vi "JTAG Function.vi"(0 "Enum":T1(ring)=enum."MULTI_ADC12_REPEAT", 1 "ARG 4":u16 format="%04x", 2 "ARG 5":u16 format="%04x", 3 "ARG 6":u16 format="%04x", 5 "ARG 1":u16 format="%04x", 7 "ARG 2":u16 format="%04x", 9 "ARG 3":u16 format="%04x", 11 "error in (no error)":errorcluster) -> (4 "ARG 7":u16 format="%04x", 8 "ARG1-ARG7":u16[](array[numeric]) format="%04x", 15 "error out":errorcluster)   [LabVIEW 2010]
panel:
  # "ARG1"
  # "ARG2"
  # "ARG3"
  # "ARG4"
  # "ARG5"
  # "ARG6"
  # "ARG7"
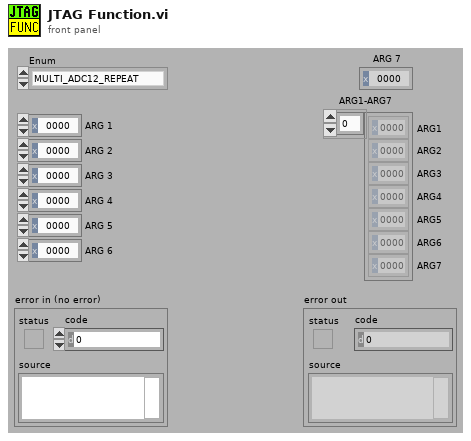
[diagram p1: front panel]
types:
  T1 = enum8{"PORT_OUT", "PORT_SEL", "PORT_RES_EN", "READ_PORT", "PORT_DIR", "SET_LCM", "PLUTO_WRITE_SINGLE", "PLUTO_READ_SINGLE", "PLUTO_WRITE_MASK", "STIM_POWER_UP", "STIM_POWER_DN", "SATURN_WRITE_SINGLE", "SATURN_READ_SINGLE", "SATURN_WRITE_BLOCK", "SATURN_READ_BLOCK", "SATURN_WRITE_MASK", "MICS_POWER_UP", "MICS_POWER_DN", "MICS_WRITE_SINGLE", "MICS_READ_SINGLE", "MICS_WRITE_BLOCK", "MICS_READ_BLOCK", "MICS_WRITE_MASK", "MEM_POWER_UP", "MEM_POWER_DN", "MEM_WRITE_SINGLE", "MEM_READ_SINGLE", "MEM_WRITE_BLOCK", "MEM_READ_BLOCK", "MEM_WRITE_MASK", "MEM_WRITE_SR", "MEM_READ_SR", "MEM_OPCODE", "INIT_VARIABLES", "DCO -> 1 MHz", "DCO -> 8 MHz", "START_STIM_CLK", "STOP_STIM_CLK", "PULSE_STIM_CLK", "PULSE_STIM_SCK", "SINGLE_ADC12", "SINGLE_ADC12_REPEAT", "MULTI_ADC12", "MULTI_ADC12_REPEAT", "Disable_ADC12", "READ_IO_VARIABLES"}
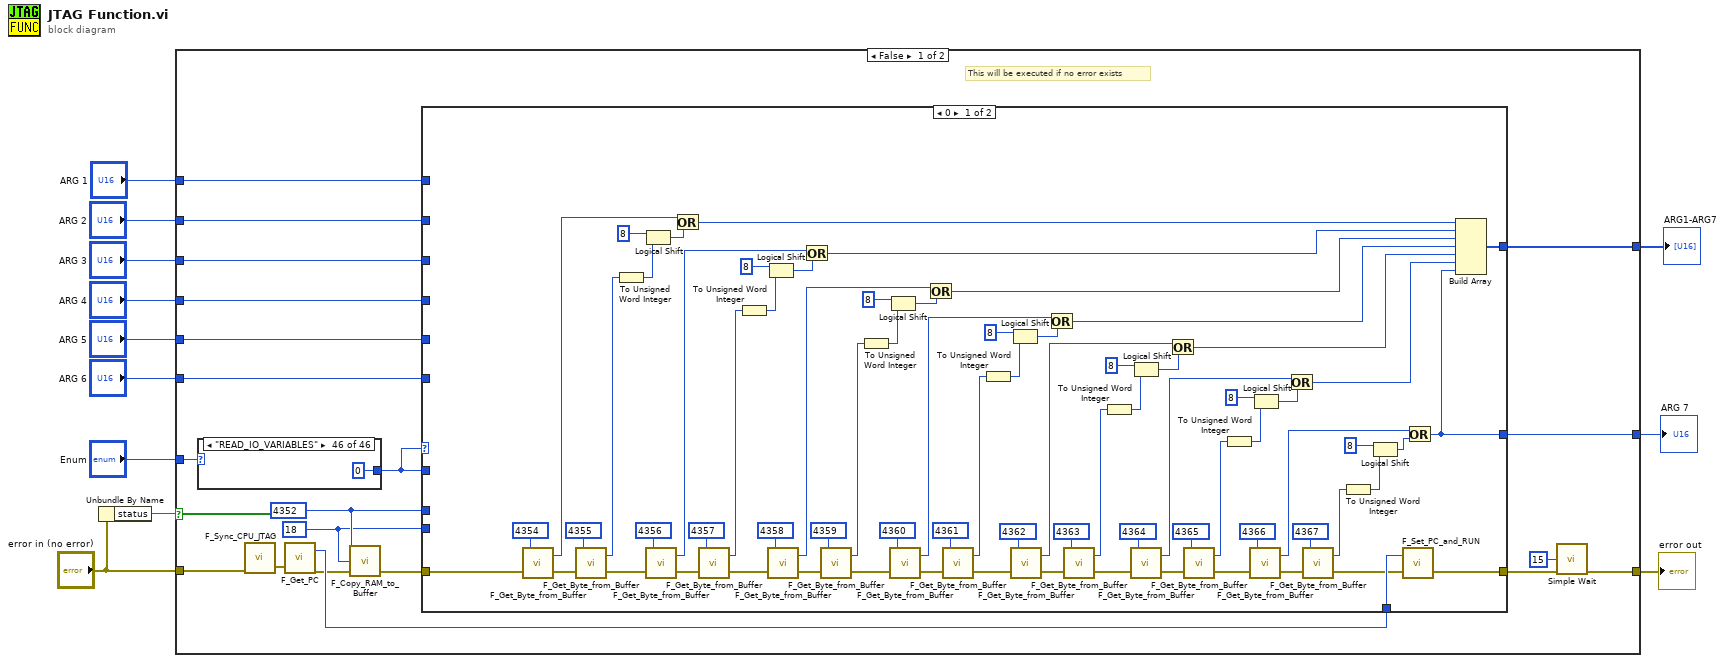
[diagram p0: block diagram]
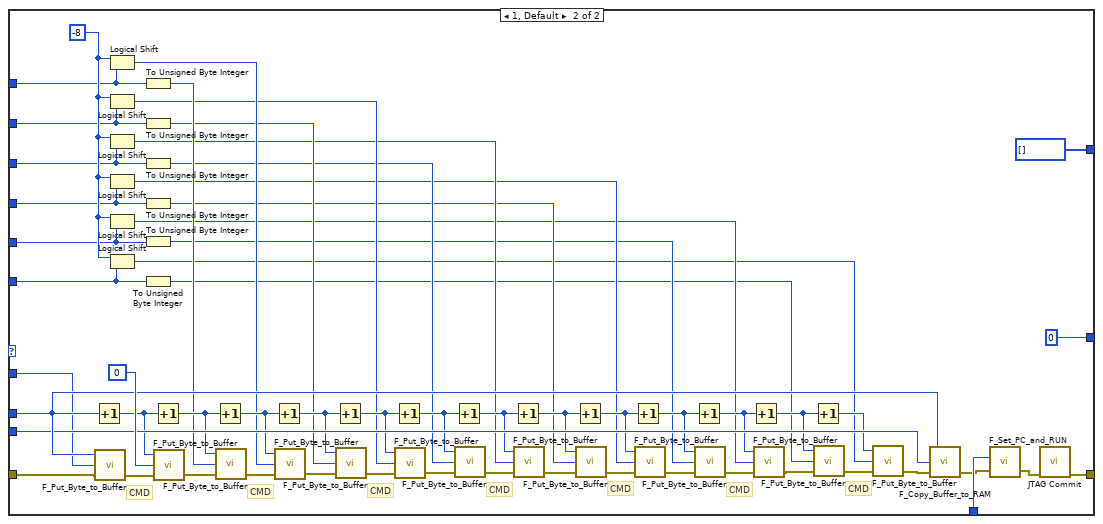
[diagram p2: hidden frame]
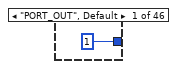
[diagram p3: hidden frame]
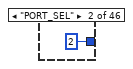
[diagram p4: hidden frame]
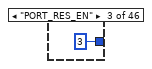
[diagram p5: hidden frame]
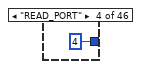
[diagram p6: hidden frame]
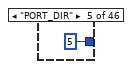
[diagram p7: hidden frame]
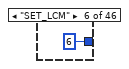
[diagram p8: hidden frame]
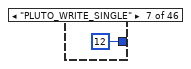
[diagram p9: hidden frame]
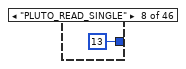
[diagram p10: hidden frame]
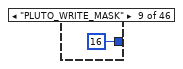
[diagram p11: hidden frame]
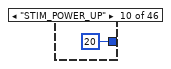
[diagram p12: hidden frame]
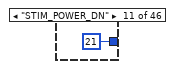
[diagram p13: hidden frame]
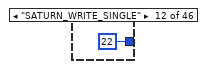
[diagram p14: hidden frame]
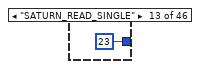
[diagram p15: hidden frame]
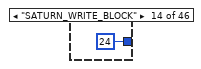
[diagram p16: hidden frame]
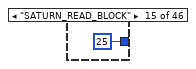
[diagram p17: hidden frame]
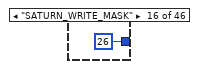
[diagram p18: hidden frame]
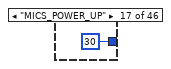
[diagram p19: hidden frame]
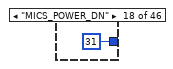
[diagram p20: hidden frame]
diagram:
  n1 = Unbundle By Name("error in (no error)") -> ("status"=w11:bool)
  n2 = case shown="False" w11 {
    tunnel: [w15 w212] -> w12
    tunnel: "error in (no error)" -> [w32 w212]
    tunnel: "Enum" -> [w26 _]
    tunnel: "ARG 6" -> [w20 _]
    tunnel: "ARG 5" -> [w21 _]
    tunnel: "ARG 4" -> [w22 _]
    tunnel: "ARG 3" -> [w23 _]
    tunnel: "ARG 2" -> [w24 _]
    tunnel: "ARG 1" -> [w25 _]
    tunnel: [w14 u16 0 ("ARG 7")] -> w2
    tunnel: [w13 u16[] []] -> w1
    frame False {
      w30 = u16 18
      w31 = u16 4352
      # "This will be executed if no error exists"
      n3 = case shown="\"READ_IO_VARIABLES\"" w26 {
        tunnel: [1 2 3 4 5 6 12 13 16 20 21 22 23 24 25 26 30 31 32 33 34 35 36 40 41 42 43 44 45 46 47 48 49 62 63 64 80 81 82 83 85 86 87 88 89 0] -> w18
        frame "PORT_OUT", Default {
        }
        frame "PORT_SEL" {
        }
        frame "PORT_RES_EN" {
        }
        frame "READ_PORT" {
        }
        frame "PORT_DIR" {
        }
        frame "SET_LCM" {
        }
        frame "PLUTO_WRITE_SINGLE" {
        }
        frame "PLUTO_READ_SINGLE" {
        }
        frame "PLUTO_WRITE_MASK" {
        }
        frame "STIM_POWER_UP" {
        }
        frame "STIM_POWER_DN" {
        }
        frame "SATURN_WRITE_SINGLE" {
        }
        frame "SATURN_READ_SINGLE" {
        }
        frame "SATURN_WRITE_BLOCK" {
        }
        frame "SATURN_READ_BLOCK" {
        }
        frame "SATURN_WRITE_MASK" {
        }
        frame "MICS_POWER_UP" {
        }
        frame "MICS_POWER_DN" {
        }
        frame "MICS_WRITE_SINGLE" {
        }
        frame "MICS_READ_SINGLE" {
        }
        frame "MICS_WRITE_BLOCK" {
        }
        frame "MICS_READ_BLOCK" {
        }
        frame "MICS_WRITE_MASK" {
        }
        frame "MEM_POWER_UP" {
        }
        frame "MEM_POWER_DN" {
        }
        frame "MEM_WRITE_SINGLE" {
        }
        frame "MEM_READ_SINGLE" {
        }
        frame "MEM_WRITE_BLOCK" {
        }
        frame "MEM_READ_BLOCK" {
        }
        frame "MEM_WRITE_MASK" {
        }
        frame "MEM_WRITE_SR" {
        }
        frame "MEM_READ_SR" {
        }
        frame "MEM_OPCODE" {
        }
        frame "INIT_VARIABLES" {
        }
        frame "DCO -> 1 MHz" {
        }
        frame "DCO -> 8 MHz" {
        }
        frame "START_STIM_CLK" {
        }
        frame "STOP_STIM_CLK" {
        }
        frame "PULSE_STIM_CLK" {
        }
        frame "PULSE_STIM_SCK" {
        }
        frame "SINGLE_ADC12" {
        }
        frame "SINGLE_ADC12_REPEAT" {
        }
        frame "MULTI_ADC12" {
        }
        frame "MULTI_ADC12_REPEAT" {
        }
        frame "Disable_ADC12" {
        }
        frame "READ_IO_VARIABLES" {
        }
      }
      n4 = call "F_Sync_CPU_JTAG.vi"("error in (no error)"=w32) -> ("error out"=w28:errorcluster)  [unwired: 1 in, 1 out]
      n5 = call "F_Get_PC.vi"("error in (no error)"=w28) -> ("error out"=w19:errorcluster, "Program Counter"=w27:u16)  [unwired: 1 in]
      n6 = call "F_Copy_RAM_to_Buffer.vi"("error in (no error)"=w19, "Block size to be copied"=w30, "RAM start address"=w31) -> ("error out"=w29:errorcluster)  [unwired: 2 in]
      n7 = case shown="0" w18 {
        tunnel: w31 -> [_ w161]
        tunnel: w30 -> [_ w160]
        tunnel: w29 -> [w59 w159]
        tunnel: w18 -> [_ w158]
        tunnel: w27 -> [w106 w157]
        tunnel: w25 -> [_ w129]
        tunnel: w24 -> [_ w128]
        tunnel: w23 -> [_ w127]
        tunnel: w22 -> [_ w126]
        tunnel: w21 -> [_ w125]
        tunnel: w20 -> [_ w124]
        tunnel: [w105 w109] -> w16
        tunnel: [w52 u16 0 ("ARG 7")] -> w14
        tunnel: [w33 u16[] []] -> w13
        frame 0 {
          n8 = call "F_Get_Byte_from_Buffer.vi"("error in (no error)"=w59, "Address of byte to be read"=u16 4354) -> ("error out"=w65:errorcluster, "Current value"=w45:u8)
          n9 = call "F_Get_Byte_from_Buffer.vi"("error in (no error)"=w65, "Address of byte to be read"=u16 4355) -> ("error out"=w53:errorcluster, "Current value"=w61:u8)
          n10 = To Unsigned Word Integer(number=w61) -> (unsigned 16bit integer=w60:u16)
          n11 = Logical Shift(y=i16 8, x=w60) -> (x << y=w51:u16)
          n12 = call "F_Get_Byte_from_Buffer.vi"("error in (no error)"=w53, "Address of byte to be read"=u16 4356) -> ("error out"=w71:errorcluster, "Current value"=w44:u8)
          n13 = Or(x=w45, y=w51) -> (x .or. y?=w34:u16)
          n14 = call "F_Get_Byte_from_Buffer.vi"("error in (no error)"=w71, "Address of byte to be read"=u16 4357) -> ("error out"=w54:errorcluster, "Current value"=w67:u8)
          n15 = To Unsigned Word Integer(number=w67) -> (unsigned 16bit integer=w66:u16)
          n16 = Logical Shift(y=i16 8, x=w66) -> (x << y=w50:u16)
          n17 = call "F_Get_Byte_from_Buffer.vi"("error in (no error)"=w54, "Address of byte to be read"=u16 4358) -> ("error out"=w77:errorcluster, "Current value"=w43:u8)
          n18 = Or(x=w44, y=w50) -> (x .or. y?=w35:u16)
          n19 = call "F_Get_Byte_from_Buffer.vi"("error in (no error)"=w77, "Address of byte to be read"=u16 4359) -> ("error out"=w55:errorcluster, "Current value"=w73:u8)
          n20 = To Unsigned Word Integer(number=w73) -> (unsigned 16bit integer=w72:u16)
          n21 = Logical Shift(y=i16 8, x=w72) -> (x << y=w49:u16)
          n22 = call "F_Get_Byte_from_Buffer.vi"("error in (no error)"=w55, "Address of byte to be read"=u16 4360) -> ("error out"=w83:errorcluster, "Current value"=w42:u8)
          n23 = Or(x=w43, y=w49) -> (x .or. y?=w36:u16)
          n24 = call "F_Get_Byte_from_Buffer.vi"("error in (no error)"=w83, "Address of byte to be read"=u16 4361) -> ("error out"=w56:errorcluster, "Current value"=w79:u8)
          n25 = To Unsigned Word Integer(number=w79) -> (unsigned 16bit integer=w78:u16)
          n26 = Logical Shift(y=i16 8, x=w78) -> (x << y=w48:u16)
          n27 = call "F_Get_Byte_from_Buffer.vi"("error in (no error)"=w56, "Address of byte to be read"=u16 4362) -> ("error out"=w89:errorcluster, "Current value"=w41:u8)
          n28 = Or(x=w42, y=w48) -> (x .or. y?=w37:u16)
          n29 = call "F_Get_Byte_from_Buffer.vi"("error in (no error)"=w89, "Address of byte to be read"=u16 4363) -> ("error out"=w57:errorcluster, "Current value"=w85:u8)
          n30 = To Unsigned Word Integer(number=w85) -> (unsigned 16bit integer=w84:u16)
          n31 = Logical Shift(y=i16 8, x=w84) -> (x << y=w47:u16)
          n32 = call "F_Get_Byte_from_Buffer.vi"("error in (no error)"=w57, "Address of byte to be read"=u16 4364) -> ("error out"=w95:errorcluster, "Current value"=w40:u8)
          n33 = Or(x=w41, y=w47) -> (x .or. y?=w38:u16)
          n34 = call "F_Get_Byte_from_Buffer.vi"("error in (no error)"=w95, "Address of byte to be read"=u16 4365) -> ("error out"=w58:errorcluster, "Current value"=w91:u8)
          n35 = To Unsigned Word Integer(number=w91) -> (unsigned 16bit integer=w90:u16)
          n36 = call "F_Get_Byte_from_Buffer.vi"("error in (no error)"=w58, "Address of byte to be read"=u16 4366) -> ("error out"=w104:errorcluster, "Current value"=w100:u8)
          n37 = Logical Shift(y=i16 8, x=w90) -> (x << y=w46:u16)
          n38 = Or(x=w40, y=w46) -> (x .or. y?=w39:u16)
          n39 = call "F_Get_Byte_from_Buffer.vi"("error in (no error)"=w104, "Address of byte to be read"=u16 4367) -> ("error out"=w103:errorcluster, "Current value"=w97:u8)
          n40 = To Unsigned Word Integer(number=w97) -> (unsigned 16bit integer=w96:u16)
          n41 = Logical Shift(y=i16 8, x=w96) -> (x << y=w98:u16)
          n42 = call "F_Set_PC_and_RUN.vi"("error in (no error)"=w103, "PC start address"=w106) -> ("error out"=w105:errorcluster)  [unwired: 1 in]
          n43 = Or(x=w100, y=w98) -> (x .or. y?=w52:u16)
          n44 = Build Array(w34, w35, w36, w37, w38, w39, w52) -> (w33:u16[])
        }
        frame 1, Default {
          w131 = -8
          # "CMD"
          # "CMD"
          # "CMD"
          # "CMD"
          # "CMD"
          # "CMD"
          # "CMD"
          n45 = Increment(x=w161) -> (x+1=w149:u16)
          n46 = call "F_Put_Byte_to_Buffer.vi"("error in (no error)"=w159, "New value"=w158, "Address of byte to be updated"=w161) -> ("error out"=w163:errorcluster)  [unwired: 2 in]
          n47 = Logical Shift(y=w131, x=w129) -> (x << y=w130:u16)
          n48 = Logical Shift(y=w131, x=w128) -> (x << y=w121:u16)
          n49 = Logical Shift(y=w131, x=w127) -> (x << y=w119:u16)
          n50 = Logical Shift(y=w131, x=w126) -> (x << y=w117:u16)
          n51 = Logical Shift(y=w131, x=w125) -> (x << y=w115:u16)
          n52 = Logical Shift(y=w131, x=w124) -> (x << y=w114:u16)
          n53 = To Unsigned Byte Integer(number=w129) -> (unsigned 8bit integer=w123:u8)
          n54 = To Unsigned Byte Integer(number=w128) -> (unsigned 8bit integer=w122:u8)
          n55 = To Unsigned Byte Integer(number=w127) -> (unsigned 8bit integer=w120:u8)
          n56 = To Unsigned Byte Integer(number=w126) -> (unsigned 8bit integer=w118:u8)
          n57 = To Unsigned Byte Integer(number=w125) -> (unsigned 8bit integer=w116:u8)
          n58 = To Unsigned Byte Integer(number=w124) -> (unsigned 8bit integer=w113:u8)
          n59 = Increment(x=w149) -> (x+1=w148:u16)
          n60 = call "F_Put_Byte_to_Buffer.vi"("error in (no error)"=w163, "New value"=u16 0, "Address of byte to be updated"=w149) -> ("error out"=w132:errorcluster)  [unwired: 2 in]
          n61 = Increment(x=w148) -> (x+1=w147:u16)
          n62 = call "F_Put_Byte_to_Buffer.vi"("error in (no error)"=w132, "New value"=w123, "Address of byte to be updated"=w148) -> ("error out"=w156:errorcluster)  [unwired: 2 in]
          n63 = Increment(x=w147) -> (x+1=w146:u16)
          n64 = call "F_Put_Byte_to_Buffer.vi"("error in (no error)"=w156, "New value"=w130, "Address of byte to be updated"=w147) -> ("error out"=w133:errorcluster)  [unwired: 2 in]
          n65 = Increment(x=w146) -> (x+1=w145:u16)
          n66 = call "F_Put_Byte_to_Buffer.vi"("error in (no error)"=w133, "New value"=w122, "Address of byte to be updated"=w146) -> ("error out"=w155:errorcluster)  [unwired: 2 in]
          n67 = Increment(x=w145) -> (x+1=w144:u16)
          n68 = call "F_Put_Byte_to_Buffer.vi"("error in (no error)"=w155, "New value"=w121, "Address of byte to be updated"=w145) -> ("error out"=w134:errorcluster)  [unwired: 2 in]
          n69 = Increment(x=w144) -> (x+1=w143:u16)
          n70 = call "F_Put_Byte_to_Buffer.vi"("error in (no error)"=w134, "New value"=w120, "Address of byte to be updated"=w144) -> ("error out"=w154:errorcluster)  [unwired: 2 in]
          n71 = Increment(x=w143) -> (x+1=w142:u16)
          n72 = call "F_Put_Byte_to_Buffer.vi"("error in (no error)"=w154, "New value"=w119, "Address of byte to be updated"=w143) -> ("error out"=w135:errorcluster)  [unwired: 2 in]
          n73 = Increment(x=w142) -> (x+1=w141:u16)
          n74 = call "F_Put_Byte_to_Buffer.vi"("error in (no error)"=w135, "New value"=w118, "Address of byte to be updated"=w142) -> ("error out"=w153:errorcluster)  [unwired: 2 in]
          n75 = Increment(x=w141) -> (x+1=w140:u16)
          n76 = call "F_Put_Byte_to_Buffer.vi"("error in (no error)"=w153, "New value"=w117, "Address of byte to be updated"=w141) -> ("error out"=w136:errorcluster)  [unwired: 2 in]
          n77 = Increment(x=w140) -> (x+1=w139:u16)
          n78 = call "F_Put_Byte_to_Buffer.vi"("error in (no error)"=w136, "New value"=w116, "Address of byte to be updated"=w140) -> ("error out"=w152:errorcluster)  [unwired: 2 in]
          n79 = Increment(x=w139) -> (x+1=w138:u16)
          n80 = call "F_Put_Byte_to_Buffer.vi"("error in (no error)"=w152, "New value"=w115, "Address of byte to be updated"=w139) -> ("error out"=w137:errorcluster)  [unwired: 2 in]
          n81 = Increment(x=w138) -> (x+1=w150:u16)
          n82 = call "F_Put_Byte_to_Buffer.vi"("error in (no error)"=w137, "New value"=w113, "Address of byte to be updated"=w138) -> ("error out"=w151:errorcluster)  [unwired: 2 in]
          n83 = call "F_Put_Byte_to_Buffer.vi"("error in (no error)"=w151, "New value"=w114, "Address of byte to be updated"=w150) -> ("error out"=w112:errorcluster)  [unwired: 2 in]
          n84 = call "F_Copy_Buffer_to_RAM.vi"("error in (no error)"=w112, "Block size to be copied"=w160, "Buffer start address"=w161) -> ("error out"=w111:errorcluster)  [unwired: 2 in]
          n85 = call "F_Set_PC_and_RUN.vi"("error in (no error)"=w111, "PC start address"=w157) -> ("error out"=w110:errorcluster)  [unwired: 1 in]
          n86 = call "JTAG Commit.vi"("error in (no error)"=w110) -> ("error out"=w109:errorcluster)  [unwired: 10 in]
        }
      }
      n87 = call "Simple Wait.vi"("mS"=u32 15, "error in"=w16) -> ("error out"=w15:errorcluster)  [unwired: 12 in, 1 out]
    }
    frame True {
      # "Error exists, skip all functions"
    }
  }
  "error out" <- w12
  "ARG 7" <- w2
  "ARG1-ARG7" <- w1
